vi "Get_LDA_+_An_data.vi"(0 "Try number":i32) -> (1 "LDA Binary output":u16[][](array[numeric])=[[142, 132, 123, 114, 103, 93, 84, 74, 65, 56, 49, 42, 35, 30, 27, 24, 23, 22, 24, 26, 30, 35, 41, 48, 56, 65, 73, 82, 93, 102, 112, 122, 132, 141, 149, 156, 164, 169, 173, 177, 180, 181, 181, 179, 176, 171, 167, 160, 153, 145, 137, 128, 118, 108, 98, 88, 79, 69, 61, 52, 45, 38, 33, 28, 25, 23, 22, 23, 25, 29, 32, 39, 45, 52, 60, 69, 78, 88, 97, 108, 118, 127, 136, 145, 153, 160, 166, 171, 176, 179, 180, 181, 180, 178, 174, 169, 164, 157, 149, 141]], 2 "Analogue Binary output":i16[][](array[numeric])=[[142, 132, 123, 114, 103, 93, 84, 74, 65, 56, 49, 42, 35, 30, 27, 24, 23, 22, 24, 26, 30, 35, 41, 48, 56, 65, 73, 82, 93, 102, 112, 122, 132, 141, 149, 156, 164, 169, 173, 177, 180, 181, 181, 179, 176, 171, 167, 160, 153, 145, 137, 128, 118, 108, 98, 88, 79, 69, 61, 52, 45, 38, 33, 28, 25, 23, 22, 23, 25, 29, 32, 39, 45, 52, 60, 69, 78, 88, 97, 108, 118, 127, 136, 145, 153, 160, 166, 171, 176, 179, 180, 181, 180, 178, 174, 169, 164, 157, 149, 141]], 3 "Block Timings":T1={"Started"=0.0, "Ended"=0.0, "Analogue Frequency Hz"=1000.0} {"Analogue Frequency Hz" format="%.2f"}, 4 "Repeat Block":bool)   [LabVIEW 2010]
doc: "The Getting Started Analog Input VI illustrates the basic concepts involved in acquiring analog input data from any data acquisition hardware.\n\nThis VI is explained in detail in the Getting Started with Analog Input section of chapter 1 of the Data Acquisition VI Reference Manual. If you are using SCXI, you should read the Getting Started with SCXI section of chapter 1 first.\n\nAfter you have installed and configured your data acquisition hardware as described in the Installation and Configuration section of chapter 1, you can run this VI to verify your hardware configuration. \n\nYou can pop-up on any front panel object for a description.\n\nIf you are using AMUX-64T boards or SCXI hardware, look at the channels control description for instructions on how to address those external channels; otherwise, you can run the VI with default inputs.\n\nOpen the diagram window to see the data acquisition VI usage."
uses:
  Controls/Block_start_and_end.ctl
  Globals/LDA_meas_global_1.vi
  Globals/LDA_meas_global_2.vi
  Globals/Meas_global.vi
panel:
  in  "milliseconds to wait":u32
  out "error out":errorcluster
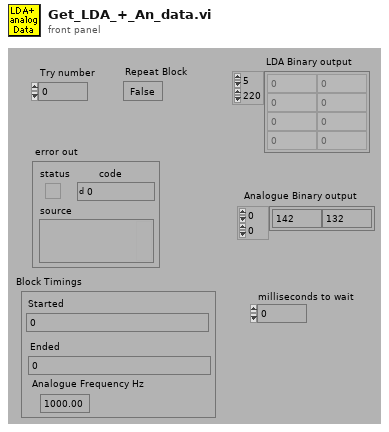
[diagram p1: front panel]
types:
  T1 = typedef "Block_start_and_end.ctl" = cluster{"Started":dbl, "Ended":dbl, "Analogue Frequency Hz":dbl}
  T2 = typedef "BSA_info_Cluster.ctl" = cluster{"GPIB Address":string, "No of Check Bytes":i32, "Extra Info":string, "COLOUR":u32, "Wavelength (nm)":dbl}
  T3 = cluster{"Burst criterion":enum16{"Envelope", "Pedestal", "Env and ped"}, "Oversize reject level":enum16{"1 (disabled)", "2", "3", "4", "5", "6", "7", "8", "9"}, "Pedestal attenuation":enum16{"0", "6", "12", "18"}, "Record length":enum16{"8", "16", "32", "64"}, "Quality factor":i16}
  T4 = typedef "Ch_and_Spans.ctl" = cluster{"high limit (10V)":sgl, "low limit (-10V)":sgl, "Ch No":i16, "Var name":string, "Use Latest Calib":bool}
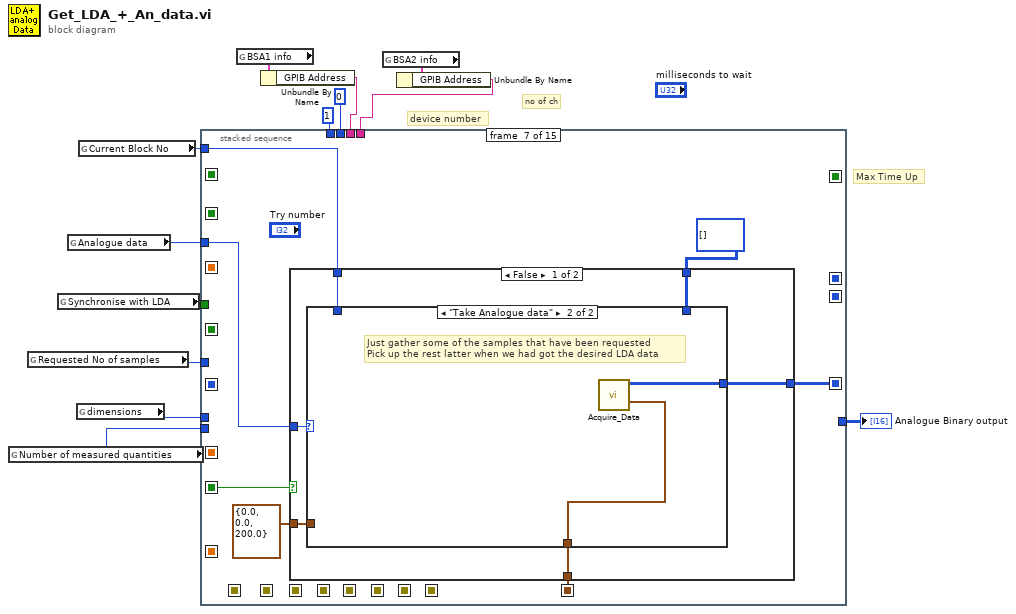
[diagram p0: block diagram]
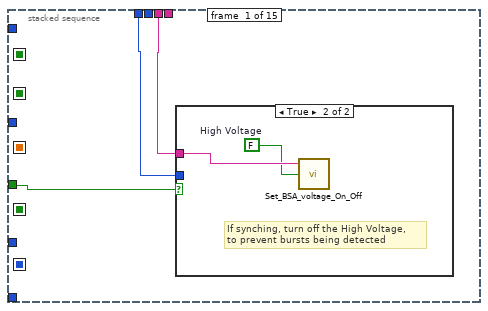
[diagram p2: hidden frame]
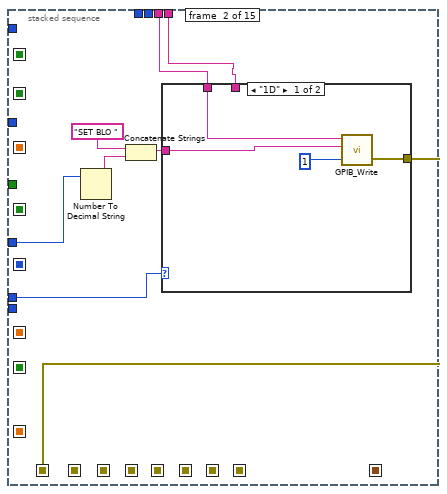
[diagram p4: hidden frame]
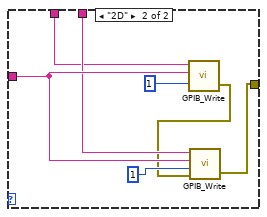
[diagram p5: hidden frame]
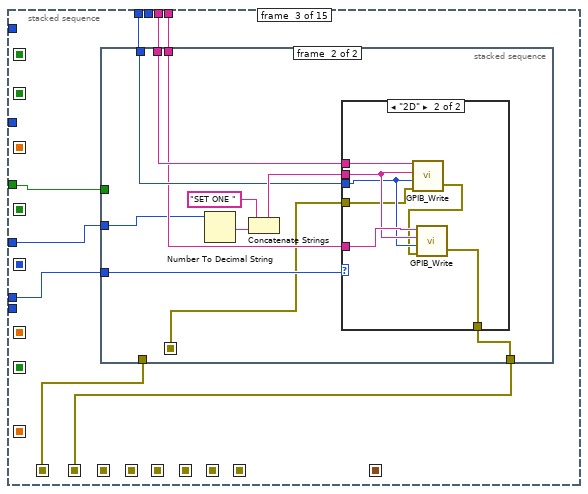
[diagram p6: hidden frame]
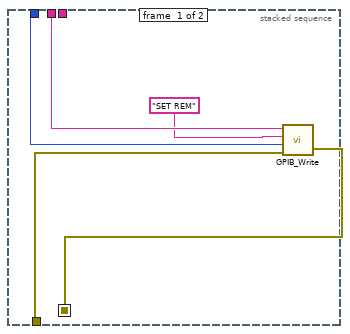
[diagram p7: hidden frame]
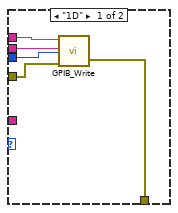
[diagram p8: hidden frame]
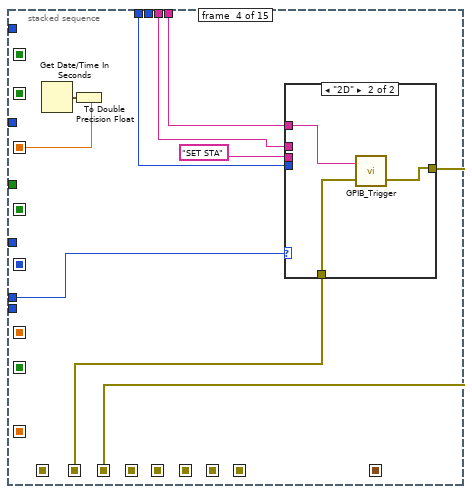
[diagram p9: hidden frame]
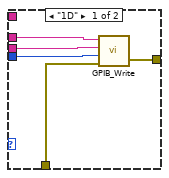
[diagram p10: hidden frame]
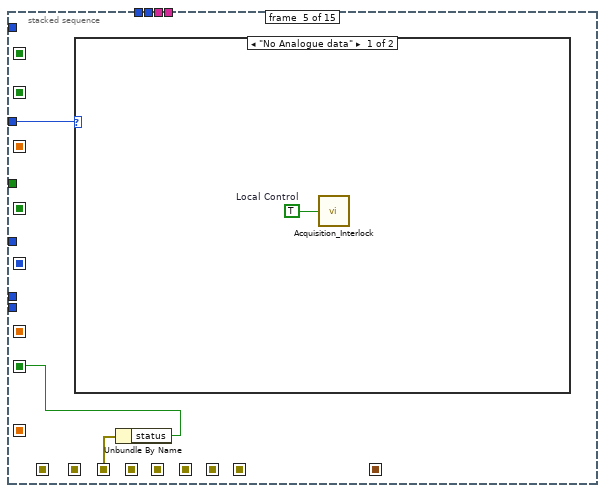
[diagram p11: hidden frame]
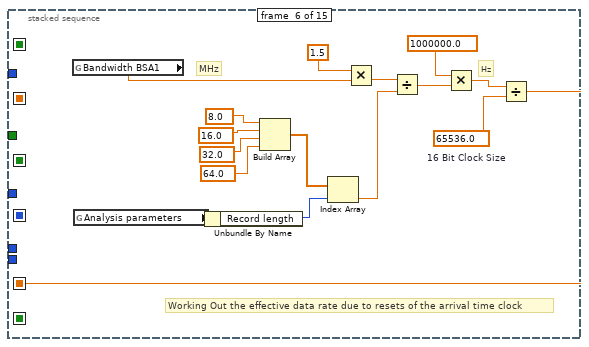
[diagram p13: hidden frame]
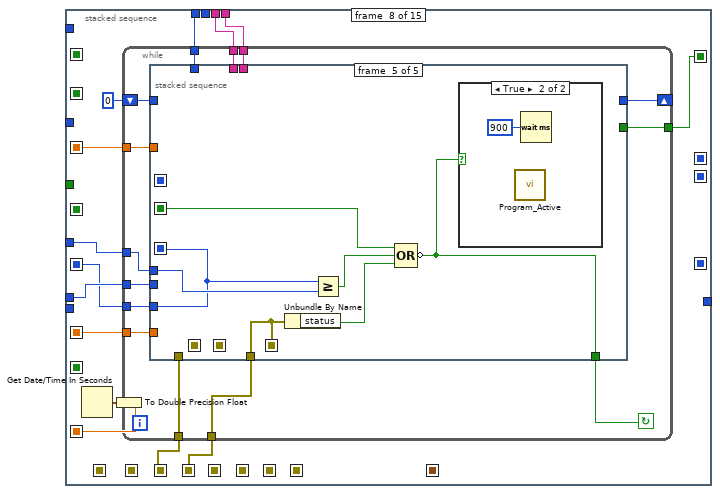
[diagram p16: hidden frame]
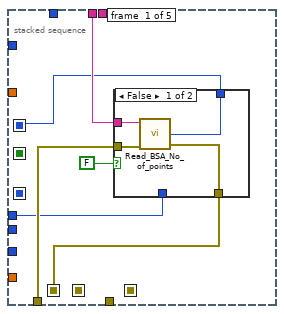
[diagram p17: hidden frame]
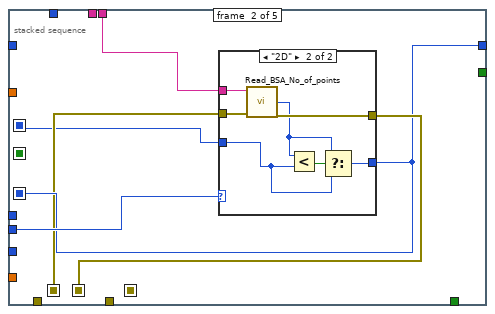
[diagram p19: hidden frame]
diagram:
  # "Max Time Up"
  # "no of ch"
  # "device number"
  n1 = global read "LDA_meas_global_1.vi" "Number of measured quantities"() -> (w11:i32)
  n2 = global read "Meas_global.vi" "Requested No of samples"() -> (w4:i32)
  n3 = global read "Meas_global.vi" "Synchronise with LDA"() -> (w3:bool)
  n4 = global read "Meas_global.vi" "Analogue data"() -> (w2:enum16{"No Analogue data", "Take Analogue data"})
  n5 = global read "Meas_global.vi" "dimensions"() -> (w6:enum16{"1D", "2D"})
  n6 = global read "Meas_global.vi" "Current Block No"() -> (w5:i32)
  n7 = global read "LDA_meas_global_1.vi" "BSA1 info"() -> (w9:T2)
  n8 = Unbundle By Name(w9) -> ("GPIB Address"=w8:string)
  n9 = global read "LDA_meas_global_2.vi" "BSA2 info"() -> (w10:T2)
  n10 = Unbundle By Name(w10) -> ("GPIB Address"=w7:string)
  n11 = stacked-sequence {
    seq-local: [_ _ _ _ _ _ _ _ _ _ w284 _ _ _ _] -> [_ _ _ _ _ _ _ _ _ _ _ _ _ w341 _]
    seq-local: [_ _ _ _ _ _ _ _ _ _ _ w298 _ _ _] -> [_ _ _ _ _ _ _ _ _ _ _ _ _ w340 _]
    seq-local: [_ _ _ _ _ _ _ _ _ _ w290 _ _ _ _] -> [_ _ _ _ _ _ _ _ _ _ _ _ _ _ w403]
    seq-local: [_ _ _ _ _ _ _ _ _ _ _ w296 _ _ _] -> [_ _ _ _ _ _ _ _ _ _ _ _ _ _ w402]
    seq-local: [_ w19 _ _ _ _ _ _ _ _ _ _ _ _ _] -> [_ _ w39 _ _ _ _ _ _ _ _ _ _ _ _]
    seq-local: [_ _ w38 _ _ _ _ _ _ _ _ _ _ _ _] -> [_ _ _ w76 _ _ _ _ _ _ _ _ _ _ _]
    seq-local: [_ _ _ w75 _ _ _ _ _ _ _ _ _ _ _] -> [_ _ _ _ w91 _ _ w138 _ _ _ _ _ _ _]
    seq-local: [_ _ _ _ _ _ _ w137 _ _ _ _ _ _ _] -> [_ _ _ _ _ _ _ _ w233 _ _ _ _ _ _]
    seq-local: [_ _ _ _ _ _ _ _ _ _ w283 _ _ _ _] -> [_ _ _ _ _ _ _ _ _ _ _ w295 _ _ _]
    seq-local: [_ _ _ _ _ _ _ _ _ _ _ w294 _ _ _] -> [_ _ _ _ _ _ _ _ _ _ _ _ w319 _ _]
    seq-local: [_ _ _ _ _ _ _ _ _ _ _ _ w318 _ _] -> [_ _ _ _ _ _ _ _ _ _ _ _ _ _ w400]
    seq-local: [_ _ _ _ _ _ _ _ _ _ _ _ _ _ w395] -> [_ _ _ _ _ _ _ _ _ _ _ _ _ _ _]
    seq-local: [_ _ _ _ _ _ _ w135 _ _ _ _ _ _ _] -> [_ _ _ _ _ _ _ _ _ _ w282 w293 _ _ _]
    seq-local: [_ _ _ _ w90 _ _ _ _ _ _ _ _ _ _] -> [_ _ _ _ _ _ w114 _ w234 _ _ _ _ _ _]
    seq-local: [_ _ _ _ _ _ _ w134 _ _ _ _ _ _ _] -> [_ _ _ _ _ _ _ _ _ w269 _ _ _ _ _]
    seq-local: [_ _ _ w74 _ _ _ _ _ _ _ _ _ _ _] -> [_ _ _ _ _ _ _ w133 _ w267 _ _ _ _ _]
    seq-local: [_ _ _ _ _ w94 _ _ _ _ _ _ _ _ _] -> [_ _ _ _ _ _ _ w131 _ _ _ _ _ _ _]
    seq-local: [_ _ _ _ _ _ _ w130 _ _ _ _ _ _ _] -> [_ _ _ _ _ _ _ _ _ _ _ _ _ _ w397]
    seq-local: [_ _ _ _ _ _ w113 _ _ _ _ _ _ _ _] -> [_ _ _ _ _ _ _ _ w231 _ _ _ _ _ _]
    seq-local: [_ _ _ _ _ _ _ _ w232 _ _ _ _ _ _] -> [_ _ _ _ _ _ _ _ _ _ w281 _ _ _ _]
    seq-local: [_ _ _ _ _ _ w111 _ _ _ _ _ _ _ _] -> [_ _ _ _ _ _ _ _ _ w265 _ _ _ _ _]
    tunnel: w11 -> [_ _ _ _ _ _ _ _ _ _ w292 w300 _ w342 _]
    tunnel: w8 -> [w15 w22 w44 w80 _ _ _ w142 _ _ w291 _ w322 _ _]
    tunnel: 0 -> [_ _ _ _ _ _ _ _ _ _ _ _ _ _ _]
    tunnel: i16 1 -> [w16 _ w45 w78 _ _ _ w132 _ _ _ _ w321 _ _]
    tunnel: w7 -> [_ w21 w42 w77 _ _ _ w139 _ _ _ w297 w320 _ _]
    tunnel: w6 -> [_ w23 w43 w81 _ _ _ w140 _ _ _ w299 w323 w336 _]
    tunnel: w5 -> [_ _ _ _ _ _ w115 _ w235 _ _ _ _ _ _]
    tunnel: w4 -> [_ w20 w41 _ _ _ _ w141 _ w270 _ _ _ _ _]
    tunnel: w3 -> [w14 _ w40 _ _ _ _ _ _ _ _ _ _ _ _]
    tunnel: w2 -> [_ _ _ _ w92 _ w116 _ w236 _ _ _ _ _ _]
    tunnel: [_ _ _ _ _ _ _ _ w230 _ _ _ _ _ _] -> w1
    frame #0 {
      n12 = case shown="True" w14 {
        tunnel: w15 -> [_ w18]
        tunnel: w16 -> [_ _]
        frame False {
        }
        frame True {
          w17 = FALSE  # High Voltage
          # "If synching, turn off the High Voltage,\nto prevent bursts being detected"
          n13 = call "Set_BSA_voltage_On_Off.vi"("GPIB address"=w18, "High Voltage"=w17) -> ()  [unwired: 1 in, 5 out]
        }
      }
    }
    frame #1 {
      n14 = Number To Decimal String(number=w20) -> (decimal integer string=w26:string)  [unwired: 1 out]
      n15 = Concatenate Strings("SET BLO ", w26) -> (w24:string)
      n16 = case shown="\"1D\"" w23 {
        tunnel: w24 -> [w28 w37]
        tunnel: w21 -> [_ w36]
        tunnel: w22 -> [w30 w35]
        tunnel: [w27 w31] -> w19
        frame "1D" {
          n17 = call "GPIB_Write.vi"("address string"=w30, "data In"=w28, "mode (0)"=i16 1) -> ("error out"=w27:errorcluster)  [unwired: 2 in, 1 out]
        }
        frame "2D" {
          n18 = call "GPIB_Write.vi"("address string"=w35, "data In"=w37, "mode (0)"=i16 1) -> ("error out"=w32:errorcluster)  [unwired: 2 in, 1 out]
          n19 = call "GPIB_Write.vi"("address string"=w36, "data In"=w37, "mode (0)"=i16 1, "error in"=w32) -> ("error out"=w31:errorcluster)  [unwired: 1 in, 1 out]
        }
      }
    }
    frame #2 {
      n20 = stacked-sequence {
        seq-local: [w46 _] -> [_ w52]
        tunnel: w45 -> [w48 w56]
        tunnel: w44 -> [w50 w55]
        tunnel: w41 -> [_ w53]
        tunnel: w43 -> [_ w57]
        tunnel: w42 -> [_ w54]
        tunnel: w40 -> [_ _]
        tunnel: w39 -> [w47 _]
        tunnel: [_ w51] -> w38
        frame #0 {
          n21 = call "GPIB_Write.vi"("address string"=w50, "data In"="SET REM", "mode (0)"=w48, "error in"=w47) -> ("error out"=w46:errorcluster)  [unwired: 1 in, 1 out]
        }
        frame #1 {
          n22 = Number To Decimal String(number=w53) -> (decimal integer string=w59:string)  [unwired: 1 out]
          n23 = Concatenate Strings("SET ONE ", w59) -> (w58:string)
          n24 = case shown="\"2D\"" w57 {
            tunnel: w55 -> [w65 w72]
            tunnel: w58 -> [w64 w70]
            tunnel: w56 -> [w63 w69]
            tunnel: w54 -> [_ w71]
            tunnel: w52 -> [w62 w68]
            tunnel: [w61 w66] -> w51
            frame "1D" {
              n25 = call "GPIB_Write.vi"("address string"=w65, "data In"=w64, "mode (0)"=w63, "error in"=w62) -> ("error out"=w61:errorcluster)  [unwired: 1 in, 1 out]
            }
            frame "2D" {
              n26 = call "GPIB_Write.vi"("address string"=w72, "data In"=w70, "mode (0)"=w69, "error in"=w68) -> ("error out"=w67:errorcluster)  [unwired: 1 in, 1 out]
              n27 = call "GPIB_Write.vi"("address string"=w71, "data In"=w70, "mode (0)"=w69, "error in"=w67) -> ("error out"=w66:errorcluster)  [unwired: 1 in, 1 out]
            }
          }
        }
      }
    }
    frame #3 {
      n28 = Get Date/Time In Seconds() -> (seconds since 1Jan1904=w73:timestamp)
      n29 = To Double Precision Float(number=w73) -> (double precision float=w74:dbl)
      n30 = case shown="\"2D\"" w81 {
        tunnel: w80 -> [w86 _]
        tunnel: "SET STA" -> [w85 _]
        tunnel: w78 -> [w84 _]
        tunnel: w77 -> [_ w89]
        tunnel: w76 -> [w83 w87]
        tunnel: [w82 w88] -> w75
        frame "1D" {
          n31 = call "GPIB_Write.vi"("address string"=w86, "data In"=w85, "mode (0)"=w84, "error in"=w83) -> ("error out"=w82:errorcluster)  [unwired: 1 in, 1 out]
        }
        frame "2D" {
          n32 = call "GPIB_Trigger.vi"("error in"=w87, "address string"=w89) -> ("error out"=w88:errorcluster)  [unwired: 1 out]
        }
      }
    }
    frame #4 {
      n33 = case shown="\"No Analogue data\"" w92 {
        frame "No Analogue data" {
          w93 = TRUE  # Local Control
          n34 = call "Acquisition_Interlock.vi"("Local Control"=w93) -> ()
        }
        frame "Take Analogue data" {
        }
      }
      n35 = Unbundle By Name(w91) -> ("status"=w90:bool)
    }
    frame #5 {
      w103 = 65536.0  # 16 Bit Clock Size
      # "Hz"
      # "MHz"
      # "Working Out the effective data rate due to resets of the arrival time clock"
      n36 = global read "LDA_meas_global_1.vi" "Bandwidth BSA1"() -> (w108:dbl)
      n37 = global read "LDA_meas_global_1.vi" "Analysis parameters"() -> (w102:T3)
      n38 = Unbundle By Name(w102) -> ("Record length"=w96:enum16{"8", "16", "32", "64"})
      n39 = Build Array(8.0, 16.0, 32.0, 64.0) -> (w97:dbl[])
      n40 = Index Array(array=w97, index=w96) -> (element=w95:dbl)
      n41 = Multiply(x=1.5, y=w108) -> (x*y=w107:dbl)
      n42 = Divide(x=w107, y=w95) -> (x/y=w106:dbl)
      n43 = Multiply(x=1000000.0, y=w106) -> (x*y=w104:dbl)
      n44 = Divide(x=w104, y=w103) -> (x/y=w94:dbl)
    }
    frame #6 {
      n45 = case shown="False" w114 {
        tunnel: w116 -> [w122 _]
        tunnel: w115 -> [w121 _]
        tunnel: [w120 w128] -> w113
        tunnel: i16[][] [] ("Binary output") -> [w119 w128]
        tunnel: [w118 w127] -> w111
        tunnel: T1 {"Started"=0.0, "Ended"=0.0, "Analogue Frequency Hz"=200.0} ("Block Timings") -> [w117 w127]
        frame False {
          n46 = case shown="\"Take Analogue data\"" w122 {
            tunnel: w121 -> [_ _]
            tunnel: [w124 w126] -> w120
            tunnel: w119 -> [w124 _]
            tunnel: [w123 w125] -> w118
            tunnel: w117 -> [w123 _]
            frame "No Analogue data" {
            }
            frame "Take Analogue data" {
              # "Just gather some of the samples that have been requested\nPick up the rest latter when we had got the desired LDA data"
              n47 = call "Acquire_Data.vi"() -> ("Binary output"=w126:i16[][], "Block Timings"=w125:T1)  [unwired: 14 out]
            }
          }
        }
        frame True {
        }
      }
    }
    frame #7 {
      n48 = Get Date/Time In Seconds() -> (seconds since 1Jan1904=w129:timestamp)
      n49 = To Double Precision Float(number=w129) -> (double precision float=w134:dbl)
      n50 = while {
        tunnel: [w143] -> w130
        tunnel: w131 -> [w144]
        tunnel: w132 -> [w145]
        tunnel: w133 -> [w146]
        tunnel: [w147] -> w135
        shift-left: 0 ("No of samples") -> [w152]
        shift-right: [w151] -> _
        tunnel: [w148] -> w137
        tunnel: w138 -> [w153]
        tunnel: w139 -> [w154]
        tunnel: w140 -> [w155]
        tunnel: w142 -> [w156]
        tunnel: w141 -> [w150]
        stop <- w149 continue-if-true
        n51 = stacked-sequence {
          seq-local: [_ w172 _ _ _] -> [_ _ _ w194 _]
          seq-local: [_ w171 _ _ _] -> [_ _ _ _ w225]
          seq-local: [w159 _ _ _ _] -> [_ w169 _ _ _]
          seq-local: [w160 _ _ _ _] -> [_ w170 _ _ _]
          seq-local: [_ _ w186 _ _] -> [_ _ _ w198 w223]
          seq-local: [_ _ _ w193 _] -> [_ _ _ _ w224]
          tunnel: w156 -> [w162 _ _ w196 _]
          tunnel: w155 -> [_ w174 _ w192 _]
          tunnel: w154 -> [_ w173 _ w197 _]
          tunnel: w153 -> [w161 _ _ _ _]
          tunnel: w152 -> [_ _ _ _ _]
          tunnel: [_ w171 _ _ _] -> w151
          tunnel: w150 -> [w158 _ w191 _ w228]
          tunnel: [_ _ _ _ w222] -> w149
          tunnel: [_ _ _ _ w224] -> w148
          tunnel: [_ _ _ _ w225] -> w147
          tunnel: w146 -> [_ _ w189 _ _]
          tunnel: w145 -> [_ _ _ w195 _]
          tunnel: w144 -> [_ _ w185 _ _]
          tunnel: [_ _ w186 _ _] -> w143
          frame #0 {
            n52 = case shown="False" FALSE {
              tunnel: w162 -> [w166 _]
              tunnel: w161 -> [w165 w167]
              tunnel: [w164 w167] -> w160
              tunnel: [w163 w168] -> w159
              tunnel: w158 -> [_ w168]
              frame False {
                n53 = call "Read_BSA_No_of_points.vi"("error in (no error)"=w165, "GPIB Address"=w166) -> ("error out"=w164:errorcluster, "No of samples"=w163:i32)  [unwired: 3 out]
              }
              frame True {
              }
            }
          }
          frame #1 {
            n54 = case shown="\"2D\"" w174 {
              tunnel: w170 -> [w176 w183]
              tunnel: w173 -> [_ w182]
              tunnel: [w176 w181] -> w172
              tunnel: w169 -> [w175 w178]
              tunnel: [w175 w177] -> w171
              frame "1D" {
              }
              frame "2D" {
                n55 = call "Read_BSA_No_of_points.vi"("error in (no error)"=w183, "GPIB Address"=w182) -> ("error out"=w181:errorcluster, "No of samples"=w179:i32)  [unwired: 3 out]
                n56 = Less?(x=w179, y=w178) -> (x < y?=w180:bool)
                n57 = Select(t=w179, s=w180, f=w178) -> (s? t:f=w177:i32)
              }
            }
          }
          frame #2 {
            n58 = Get Date/Time In Seconds() -> (seconds since 1Jan1904=w184:timestamp)
            n59 = To Double Precision Float(number=w184) -> (double precision float=w190:dbl)
            n60 = Subtract(x=w190, y=w189) -> (x-y=w188:dbl)
            n61 = Divide(x=w191, y=w185) -> (x/y=w187:dbl)
            n62 = Greater?(x=w188, y=w187) -> (0:w186:bool)
          }
          frame #3 {
            n63 = case shown="True" w198 {
              tunnel: w197 -> [_ w200]
              tunnel: w196 -> [_ w208]
              tunnel: w195 -> [_ w207]
              tunnel: w194 -> [w199 w206]
              tunnel: [w199 w202] -> w193
              tunnel: w192 -> [_ w205]
              frame False {
              }
              frame True {
                n64 = case shown="\"2D\"" w205 {
                  tunnel: w207 -> [w213 w218]
                  tunnel: "SET IDL" -> [w214 w219]
                  tunnel: w208 -> [w210 w220]
                  tunnel: w200 -> [_ w221]
                  tunnel: w206 -> [w211 w217]
                  tunnel: [w212 w215] -> w204
                  frame "1D" {
                    n65 = call "GPIB_Write.vi"("address string"=w210, "data In"=w214, "mode (0)"=w213, "error in"=w211) -> ("error out"=w212:errorcluster)  [unwired: 1 in, 1 out]
                  }
                  frame "2D" {
                    n66 = call "GPIB_Write.vi"("address string"=w220, "data In"=w219, "mode (0)"=w218, "error in"=w217) -> ("error out"=w216:errorcluster)  [unwired: 1 in, 1 out]
                    n67 = call "GPIB_Write.vi"("address string"=w221, "data In"=w219, "mode (0)"=w218, "error in"=w216) -> ("error out"=w215:errorcluster)  [unwired: 1 in, 1 out]
                  }
                }
                n68 = Bundle By Name(cluster=w204, "status"=TRUE ("Bundle Element"), "source"="Max Time in block exceeded, BSA's have been set to idle and the program should now move onto the next measurement position" ("Bundle Element")) -> (w202:errorcluster)
              }
            }
          }
          frame #4 {
            n69 = Unbundle By Name(w224) -> ("status"=w226:bool)
            n70 = Greater Or Equal?(x=w225, y=w228) -> (x >= y?=w227:bool)
            n71 = Compound Arithmetic op=OR(w223, w227, w226) -> (invert w222:bool)
            n72 = case shown="True" w222 {
              frame False {
              }
              frame True {
                n73 = call "Program_Active.vi"() -> ()  [unwired: 1 in]
                n74 = Wait (ms)(milliseconds to wait=u32 900) -> ()  [unwired: 1 out]
              }
            }
          }
        }
      }
    }
    frame #8 {
      n75 = case shown="False" w234 {
        tunnel: w236 -> [w242 _]
        tunnel: w235 -> [w241 _]
        tunnel: w233 -> [w240 w263]
        tunnel: [w239 w263] -> w232
        tunnel: w231 -> [w238 w262]
        tunnel: [w237 w262] -> w230
        frame False {
          n76 = case shown="\"Take Analogue data\"" w242 {
            tunnel: w241 -> [_ _]
            tunnel: w240 -> [w244 w254]
            tunnel: [w244 w252] -> w239
            tunnel: w238 -> [w243 w251]
            tunnel: [w243 w249] -> w237
            frame "No Analogue data" {
            }
            frame "Take Analogue data" {
              w255 = u8 8  # unsigned 8bit integer
              # "Number of Unread samples"
              n77 = global read "Meas_global.vi" "Ch & spans + mod limits"() -> (w245:T4[])
              n78 = call "ADC488_Manual_tl.vi"("GPIB Address"=w255, "Command String"="U5", "Byte Count Requested"=500, "error in (no error)"=w254) -> ("Response String"=w258:string, "error out"=w253:errorcluster)  [unwired: 3 in, 7 out]
              n79 = Decimal String To Number(string=w258) -> (number=w247:i32)  [unwired: 3 out]
              n80 = call "Add_dummy_channels.vi"("Ch & spans"=w245) -> ("Ch & spans"=w246:T4[])
              n81 = call "Make_Odd.vi"("No of samples"=w247) -> ("Odd No of Samples"=w248:i32)
              n82 = call "ADC_Read.vi"("GPIB Address"=w255, "Ch & spans"=w246, "number of scans to read"=w248, "error in (no error)"=w253) -> ("binary data"=w250:i16[][], "error out"=w252:errorcluster)  [unwired: 1 in, 9 out]
              n83 = for {
                tunnel: w251 -> [w261] mode=indexing
                tunnel: w250 -> [w260] mode=indexing
                tunnel: [w259] -> w249 mode=indexing
                n84 = Build Array (concatenate)(w261, w260) -> (w259:i16[])
              }
            }
          }
        }
        frame True {
        }
      }
    }
    frame #9 {
      n85 = global read "Meas_global.vi" "Remote control"() -> (w271:bool)
      n86 = Get Date/Time In Seconds() -> (seconds since 1Jan1904=w264:timestamp)
      n87 = To Double Precision Float(number=w264) -> (double precision float=w266:dbl)
      n88 = case shown="True" w271 {
        tunnel: w270 -> [_ w280]
        tunnel: w269 -> [_ w276]
        tunnel: w266 -> [_ w272]
        frame False {
        }
        frame True {
          n89 = global read "Meas_global.vi" "Actual Sampling rate (Hz)"() -> (w279:dbl)
          n90 = Divide(x=w279, y=sgl 1.3) -> (x/y=w277:dbl)
          n91 = Divide(x=w280, y=w277) -> (x/y=w275:dbl)
          n92 = Subtract(x=w272, y=w276) -> (x-y=w274:dbl)
          n93 = Subtract(x=w275, y=w274) -> (x-y=w273:dbl)
          n94 = call "Wait_seconds.vi"("Seconds to wait"=w273) -> ()
        }
      }
      n95 = Bundle By Name(cluster=w265, "Started"=w267, "Ended"=w266) -> (→"Block Timings":T1)
    }
    frame #10 {
      n96 = global read "LDA_meas_global_1.vi" "BSA1 info"() -> (w286:T2)
      n97 = Unbundle By Name(w286) -> ("No of Check Bytes"=w285:i32)
      n98 = Multiply(x=w282, y=2) -> (x*y=w288:i32)
      n99 = Multiply(x=w288, y=w292) -> (x*y=w287:i32)
      n100 = call "Read_BSA_data.vi"("GPIB Address"=w291, "No of Check Bytes"=w285, "Bytes per block"=w287, "error in (no error)"=w281) -> ("transmission okay"=w290:bool, "array of velocity data"=w284:u16[], "error out"=w283:errorcluster)  [unwired: 9 out]
    }
    frame #11 {
      n101 = case shown="\"1D\"" w299 {
        tunnel: [w303 w312] -> w298
        tunnel: w297 -> [_ w311]
        tunnel: w300 -> [_ w316]
        tunnel: w293 -> [_ w313]
        tunnel: [TRUE ("transmission okay") w307] -> w296
        tunnel: w295 -> [w301 w306]
        tunnel: [w301 w305] -> w294
        frame "1D" {
          n102 = Build Array(u16 0) -> (w303:u16[])
        }
        frame "2D" {
          n103 = global read "LDA_meas_global_2.vi" "BSA2 info"() -> (w308:T2)
          n104 = Unbundle By Name(w308) -> ("No of Check Bytes"=w310:i32)
          n105 = Multiply(x=w313, y=2) -> (x*y=w315:i32)
          n106 = Multiply(x=w315, y=w316) -> (x*y=w309:i32)
          n107 = call "Read_BSA_data.vi"("GPIB Address"=w311, "No of Check Bytes"=w310, "Bytes per block"=w309, "error in (no error)"=w306) -> ("transmission okay"=w307:bool, "array of velocity data"=w312:u16[], "error out"=w305:errorcluster)  [unwired: 9 out]
        }
      }
    }
    frame #12 {
      n108 = case shown="\"2D\"" w323 {
        tunnel: w321 -> [w326 w332]
        tunnel: "SET LOC" -> [w327 w333]
        tunnel: w320 -> [_ w334]
        tunnel: w322 -> [w328 w335]
        tunnel: w319 -> [w325 w331]
        tunnel: [w324 w329] -> w318
        frame "1D" {
          n109 = call "GPIB_Write.vi"("address string"=w328, "data In"=w327, "mode (0)"=w326, "error in"=w325) -> ("error out"=w324:errorcluster)  [unwired: 1 in, 1 out]
        }
        frame "2D" {
          n110 = call "GPIB_Write.vi"("address string"=w334, "data In"=w333, "mode (0)"=w332, "error in"=w331) -> ("error out"=w330:errorcluster)  [unwired: 1 in, 1 out]
          n111 = call "GPIB_Write.vi"("address string"=w335, "data In"=w333, "mode (0)"=w332, "error in"=w330) -> ("error out"=w329:errorcluster)  [unwired: 1 in, 1 out]
        }
      }
    }
    frame #13 {
      n112 = case shown="3.." w342 {
        tunnel: w341 -> [_ w350 w359 w375]
        tunnel: w340 -> [_ w349 w374 w394]
        tunnel: [w347 w358 w373 w393] -> w339
        tunnel: [w347 w357 w372 w392] -> w338
        frame ..0 {
          w348 = u16 0
          n113 = Initialize Array(w348, w348, w348) -> (w347:u16[][])
        }
        frame 1 {
          n114 = Array Size(array=w349) -> (size(s)=w356:i32)
          n115 = Array Size(array=w350) -> (size(s)=w351:i32)
          n116 = To Unsigned Word Integer(number=w356) -> (unsigned 16bit integer=w355:u16)
          n117 = To Unsigned Word Integer(number=w351) -> (unsigned 16bit integer=w352:u16)
          n118 = Build Array (concatenate)(w355, w349) -> (w354:u16[])
          n119 = Build Array (concatenate)(w352, w350) -> (w353:u16[])
          n120 = Build Array(w353) -> (w358:u16[][])
          n121 = Build Array(w354) -> (w357:u16[][])
        }
        frame 2 {
          n122 = Decimate 1D Array(w374) -> (w371:u16[], w369:u16[])
          n123 = Decimate 1D Array(w359) -> (w360:u16[], w362:u16[])
          n124 = Array Size(array=w371) -> (size(s)=w370:i32)
          n125 = Array Size(array=w360) -> (size(s)=w361:i32)
          n126 = To Unsigned Word Integer(number=w370) -> (unsigned 16bit integer=w368:u16)
          n127 = To Unsigned Word Integer(number=w361) -> (unsigned 16bit integer=w363:u16)
          n128 = Build Array (concatenate)(w368, w371) -> (w367:u16[])
          n129 = Build Array (concatenate)(w368, w369) -> (w366:u16[])
          n130 = Build Array (concatenate)(w363, w360) -> (w364:u16[])
          n131 = Build Array (concatenate)(w363, w362) -> (w365:u16[])
          n132 = Build Array(w367, w366) -> (w372:u16[][])
          n133 = Build Array(w364, w365) -> (w373:u16[][])
        }
        frame 3.. {
          n134 = Decimate 1D Array(w394) -> (w391:u16[], w389:u16[], w388:u16[])
          n135 = Decimate 1D Array(w375) -> (w376:u16[], w378:u16[], w379:u16[])
          n136 = Array Size(array=w391) -> (size(s)=w390:i32)
          n137 = Array Size(array=w376) -> (size(s)=w377:i32)
          n138 = To Unsigned Word Integer(number=w390) -> (unsigned 16bit integer=w387:u16)
          n139 = To Unsigned Word Integer(number=w377) -> (unsigned 16bit integer=w380:u16)
          n140 = Build Array (concatenate)(w387, w391) -> (w386:u16[])
          n141 = Build Array (concatenate)(w387, w389) -> (w385:u16[])
          n142 = Build Array (concatenate)(w387, w388) -> (w384:u16[])
          n143 = Build Array (concatenate)(w380, w376) -> (w381:u16[])
          n144 = Build Array (concatenate)(w380, w378) -> (w382:u16[])
          n145 = Build Array (concatenate)(w380, w379) -> (w383:u16[])
          n146 = Build Array(w386, w385, w384) -> (w392:u16[][])
          n147 = Build Array(w381, w382, w383) -> (w393:u16[][])
        }
      }
      n148 = case shown="\"2D\"" w336 {
        tunnel: w339 -> [w343 w346]
        tunnel: w338 -> [_ w345]
        tunnel: [w343 w344] -> w337
        frame "1D" {
        }
        frame "2D" {
          n149 = Build Array (concatenate)(w346, w345) -> (w344:u16[][])
        }
      }
      "LDA Binary output" <- w337
    }
    frame #14 {
      w401 = FALSE  # Dialog Box
      n150 = Unbundle By Name(w400) -> ("status"=w395:bool)
      n151 = Compound Arithmetic op=AND(w403, w402, invert w395) -> (invert w398:bool)
      n152 = call "EnFlo_Error_Handler.vi"("error in (no error)"=w400, "Error Type"="BSA Comms Error", "Dialog Box (T)"=w401) -> ()  [unwired: 3 out]
      n153 = Compound Arithmetic op=AND(invert w397, w398) -> (→"Repeat Block":bool)
      "error out" <- w400
    }
  }
  "Analogue Binary output" <- w1
